vi "Decimate DFD (SANDBOX).vi"(8 "error in (no error)":errorcluster, 10 "Decimation Factor":i32, 11 "Waveforms in":waveform(dbl)[](array[waveform])) -> (0 "error out":errorcluster, 3 "waveforms out":waveform(dbl)[](array[waveform]))   [LabVIEW 2019, in "Instrument.Lockin.lvlib" / "Instrument.DAQ.lvclass"]
uses:
  <vilib>/addons/Digital Filter Design/_Objects.llb/DFD Multirate Filtering Mode.ctl
  <vilib>/Analysis/2dsp.llb/Decimate (single shot, DBL).vi
  Instrument.DAQ.lvclass
  <vilib>/addons/Digital Filter Design/NI_DigFilterLicensed.lvlib
  <vilib>/addons/Digital Filter Design/_Objects.llb/DFD Multirate Filter Specification (Design).ctl
  <vilib>/Analysis/NI_AALPro.lvlib
  <vilib>/measure/NI_MAPro.lvlib
  <vilib>/addons/Digital Filter Design/_Objects.llb/DFD Filter Ripple Specification (Design).ctl
  <vilib>/measure/maresamp.llb/Resample N Waveforms (continuous).vi
  <vilib>/addons/Digital Filter Design/Multirate.llb/DFD NStage MRate Filtering for Single Block (Wfm).vi
  <vilib>/addons/Digital Filter Design/Multirate.llb/DFD NStage MRate Filtering (Wfm).vi
  <vilib>/addons/Digital Filter Design/Multirate.llb/DFD MRate Filtering for Single Block (Wfm NChan).vi
panel:
  out "x != y?":bool
  out "x/y":dbl
  out "Magnitude Response":cluster{"f0":dbl, "df":dbl, "values":dbl[]}[](graph)
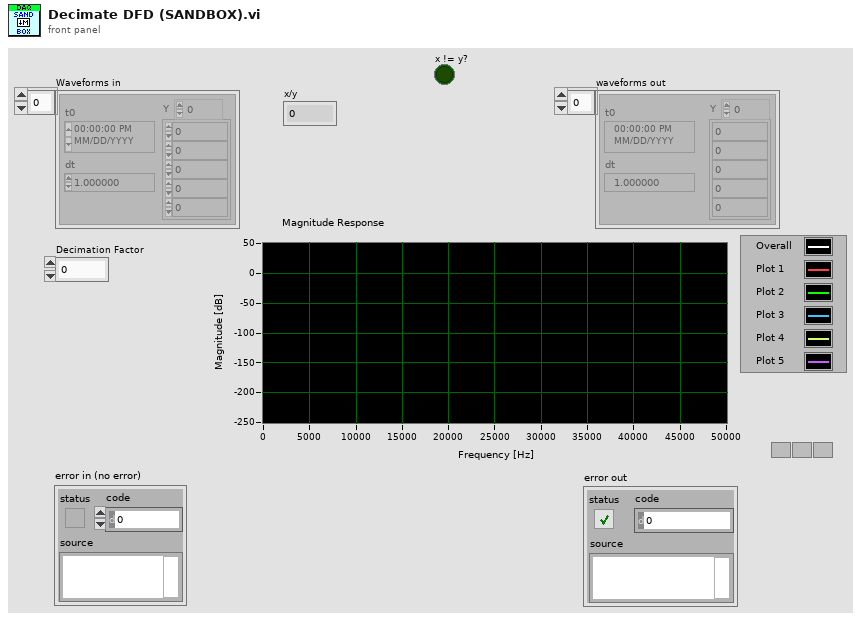
[diagram p1: front panel]
types:
  T1 = typedef "NI_DigFilterLicensed.lvlib/DFD Multirate Filtering Mode.ctl" = u16
  T2 = typedef "NI_DigFilterLicensed.lvlib/DFD Filter Ripple Specification (Design).ctl" = cluster{"passband":dbl, "stopband":dbl, "dB/linear? (T: dB)":bool}
  T3 = typedef "NI_DigFilterLicensed.lvlib/DFD Multirate Filter Specification (Design).ctl" = cluster{"fpass":dbl, "fstop":dbl}
  T4 = typedef "NI_DigFilterLicensed.lvlib/DFD Multirate Filter Obj.ctl" = cluster{"mMRate_Structure":enum16{"CIC", "FIR", "IIR", "Lattice"}, "mMRate_Mode":T5, "mMRate_Factor":i32, "mMRate_FIRParams":cluster{"mMRate_FIR_H":dbl[], "mMRate_FIR_IsNyquist?":bool, "mMRate_FIR_IsSymmetric?":bool}, "mMRate_CICParams":cluster{"mMRate_CIC_#Stage":i32, "mMRate_CIC_Lag":i32, "mMRate_CIC_Type":enum16{"Lowpass", "Highpass"}}, "mMRate_Order":i32, "mMRate_Version":string, "mMRate_Comments":string, "mMRate_RationalFactor":cluster{"mMRate_L":i32, "mMRate_M":i32}, "mMRate_Fs":dbl, "mMRate_Quantized?":bool, "mMRate_QFilterGain":dbl, "mMRate_CoefWl":i16, "mMRate_Scaling":cluster{"mMRate_ScaleByPowerOf2?":bool, "mMRate_ScaleType":T6}, "mMRate_InputWl":i16, "mMRate_OutputWl":i16, "mMRate_OutputMode":T7, "mMRate_MultMode":T8, "mMRate_BitPruning":bool, "mMRate_GainWl":i16, "mMRate_OutputFwl":i16, "mMRate_SumIwl":i16, "mMRate_InputIwl ":i16, "mMRate_SumWl":i16, "mMRate_CoefIwl":i16}
  T5 = typedef "NI_DigFilterLicensed.lvlib/DFD Multirate Mode.ctl" = i16
  T6 = typedef "NI_DigFilterLicensed.lvlib/DFD Coef Norm Type.ctl" = enum16{"No Norm", "Time Domain 1-Norm", "Time Domain 2-Norm", "Time Domain Inf-Norm"}
  T7 = typedef "NI_DigFilterLicensed.lvlib/DFD Round-off Mode.ctl" = enum16{"Nearest", "Truncation"}
  T8 = typedef "NI_DigFilterLicensed.lvlib/DFD FXP MRate Multiply Mode.ctl" = enum16{"Truncated", "Full"}
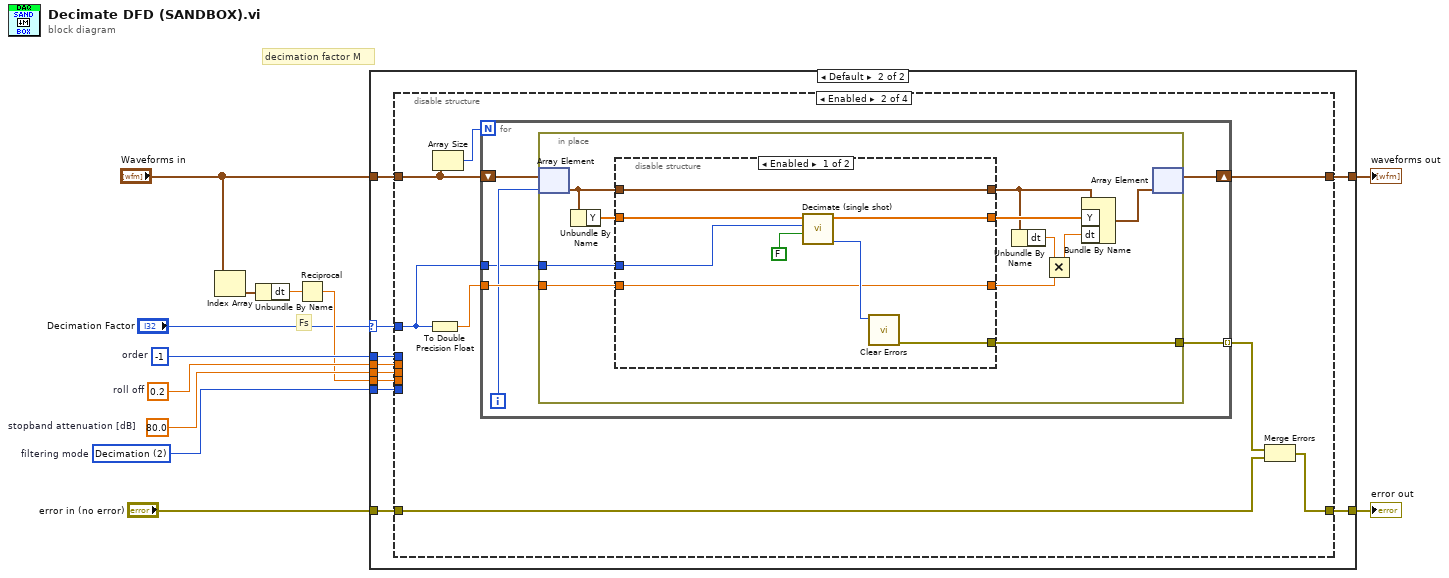
[diagram p0: block diagram]
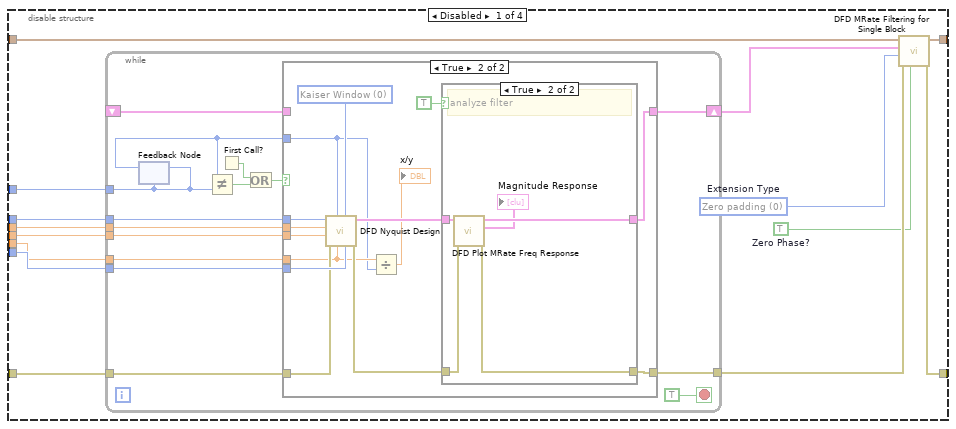
[diagram p3: hidden frame]
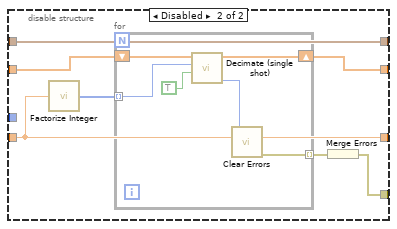
[diagram p6: hidden frame]
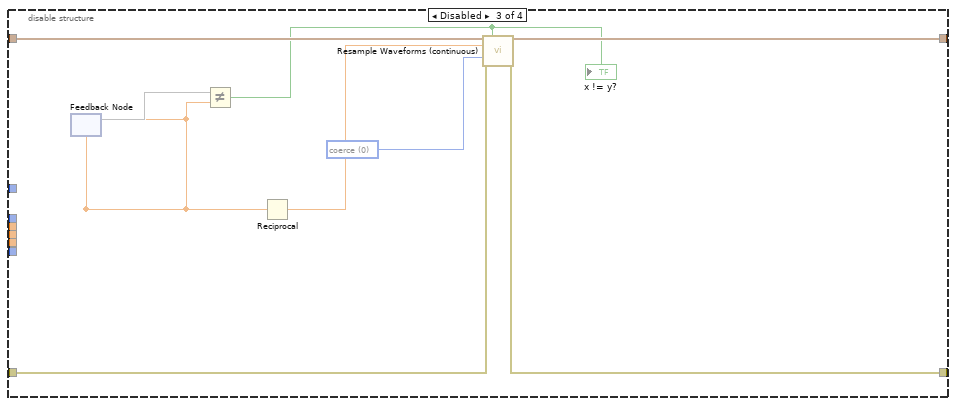
[diagram p7: hidden frame]
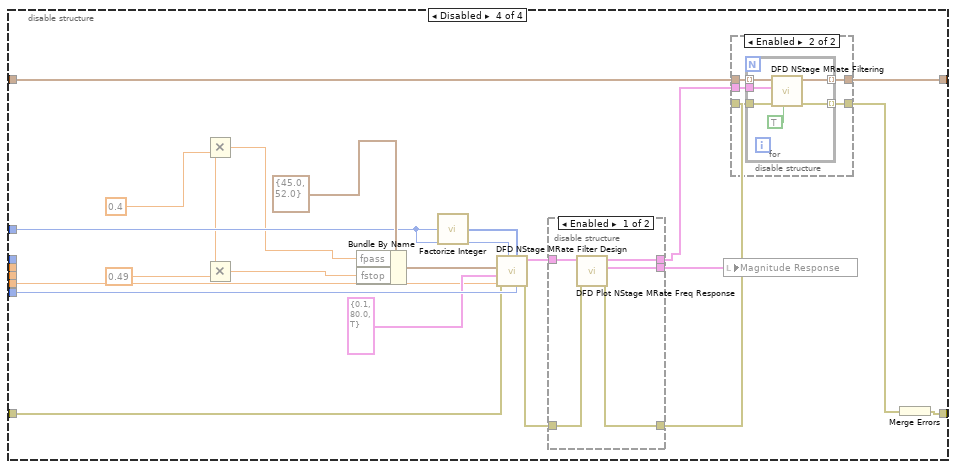
[diagram p8: hidden frame]
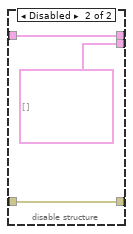
[diagram p9: hidden frame]
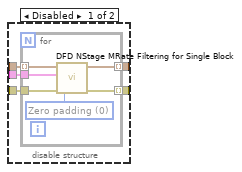
[diagram p10: hidden frame]
diagram:
  w11 = -1  # order
  w9 = 80.0  # stopband attenuation [dB]
  w10 = T1 2 items=["No Rate Change", "Interpolation", "Decimation"]  # filtering mode
  w12 = 0.2  # roll off
  # "Fs"
  # "decimation factor M"
  n1 = Index Array(array="Waveforms in") -> (element=w7:waveform(dbl))  [unwired: 1 in]
  n2 = Unbundle By Name(w7) -> ("dt"=w3:dbl)
  n3 = Reciprocal(x=w3) -> (1/x=w2:dbl)
  n4 = case shown="Default" "Decimation Factor" {
    selector: "Decimation Factor" -> [_ w18]
    tunnel: w12 -> [_ w24]
    tunnel: w10 -> [_ w23]
    tunnel: w9 -> [_ w22]
    tunnel: w11 -> [_ w21]
    tunnel: "Waveforms in" -> [w14 w17]
    tunnel: [w14 w20] -> w8
    tunnel: w2 -> [_ w19]
    tunnel: [w13 w16] -> w5
    tunnel: "error in (no error)" -> [w13 w15]
    frame 0, 1 {
    }
    frame Default {
      n5 = disable-structure shown="Enabled" {
        disable-tunnel: w24 -> [w38 _ _ _]
        disable-tunnel: w23 -> [w37 _ _ w152]
        disable-tunnel: w22 -> [w36 _ _ _]
        disable-tunnel: w21 -> [w35 _ _ _]
        disable-tunnel: [w34 w82 w130 w151] -> w20
        disable-tunnel: w19 -> [w33 _ _ w132]
        disable-tunnel: w17 -> [w30 w80 w131 w135]
        disable-tunnel: w18 -> [w29 w77 _ w143]
        disable-tunnel: [w28 w83 w128 w144] -> w16
        disable-tunnel: w15 -> [w25 w84 w129 w147]
        frame Disabled {
          w26 = TRUE  # Zero Phase?
          w27 = u16 0 items=["Zero padding", "Symmetric", "Periodic"]  # Extension Type
          n6 = while {
            tunnel: w38 -> [w53]
            tunnel: w37 -> [w52]
            tunnel: w36 -> [w51]
            tunnel: w35 -> [w50]
            tunnel: w33 -> [w49]
            tunnel: [w47] -> w31
            shift-right: [w48] -> w32
            shift-left: _ -> [w45]
            tunnel: w29 -> [w40]
            tunnel: w25 -> [w41]
            stop <- TRUE stop-if-true
            n7 = feedback #1(w40) -> (w39:i32)
            n8 = feedback-in #1(w40) -> ()
            n9 = Not Equal?(x=w39, y=w40) -> (x != y?=w43:bool)
            n10 = First Call?() -> (First Call?: T/F=w44:bool)
            n11 = Or(x=w44, y=w43) -> (x .or. y?=w42:bool)
            n12 = case shown="True" w42 {
              tunnel: w53 -> [_ w69]
              tunnel: w52 -> [_ w68]
              tunnel: w51 -> [_ w67]
              tunnel: w50 -> [_ w66]
              tunnel: w49 -> [_ w58]
              tunnel: [w54 w63] -> w48
              tunnel: [w55 w62] -> w47
              tunnel: w45 -> [w54 _]
              tunnel: w39 -> [_ w57]
              tunnel: w41 -> [w55 w59]
              frame False {
              }
              frame True {
                w65 = u16 0 items=["Kaiser Window", "Dolph-Chebyshev Window", "Equi-Ripple", "Positive Equi-Ripple"] ("method")
                n13 = call <vilib>:"DFD Nyquist Design.vi"("filtering mode"=w68, "method"=w65, "fs in [Hz]"=w58, "factor"=w57, "error in (no error)"=w59, "stopband attenuation [dB]"=w67, "roll off"=w69, "order"=w66) -> ("error out"=w60:errorcluster, "multirate filter out"=w64:T4)  [unwired: 2 out]
                n14 = Divide(x=w58, y=w57) -> (x/y=→"x/y":dbl)
                n15 = case shown="True" TRUE {
                  tunnel: w64 -> [w71 w76]
                  tunnel: w60 -> [w70 w73]
                  tunnel: [w71 w75] -> w63
                  tunnel: [w70 w72] -> w62
                  frame False {
                  }
                  frame True {
                    # "analyze filter"
                    n16 = call <vilib>:"DFD Plot MRate Freq Response.vi"("error in (no error)"=w73, "multirate filter in"=w76) -> ("error out"=w72:errorcluster, "magnitude response"=→"Magnitude Response":cluster{"f0":dbl, "df":dbl, "values":dbl[]}[], "multirate filter out"=w75:T4)  [unwired: 5 in, 2 out]
                  }
                }
              }
            }
          }
          n17 = call-poly <vilib>:"DFD MRate Filtering for Single Block.vi"("zero phase? (T)"=w26, "error in (no error)"=w31, "extension type"=w27, "multirate filter"=w32, "signal in"=w30) -> ("error out"=w28:errorcluster, "signal out"=w34:waveform(dbl)[])  [unwired: 5 out]
        }
        frame Enabled {
          n18 = To Double Precision Float(number=w77) -> (double precision float=w78:dbl)
          n19 = Array Size(array=w80) -> (size(s)=w79:i32)
          n20 = for {
            N: w79 -> [_]
            tunnel: w78 -> [w90]
            tunnel: [w89] -> w81 mode=indexing
            shift-right: [w86] -> w82
            shift-left: w80 -> [w88]
            tunnel: w77 -> [w85]
            i -> [w87]
            n21 = in-place {
              in-place-border: w90 -> [w100]
              in-place-border: [w99] -> w89
              in-place-border: w85 -> [w91]
              n22 = in-place-array #2(w88, w87) -> (w93:waveform(dbl))
              n23 = Unbundle By Name(w93) -> ("Y"=w101:dbl[])
              n24 = disable-structure shown="Enabled" {
                disable-tunnel: w101 -> [w109 w116]
                disable-tunnel: w93 -> [w105 w112]
                disable-tunnel: [w105 w112] -> w97
                disable-tunnel: w100 -> [w103 w110]
                disable-tunnel: [w107 w113] -> w99
                disable-tunnel: [w104 w111] -> w98
                disable-tunnel: [w103 w110] -> w95
                disable-tunnel: w91 -> [w102 _]
                frame Enabled {
                  n25 = call-poly <vilib>:"Decimate (single shot).vi"("averaging"=FALSE, "decimating factor"=w102, "X"=w109) -> ("error"=w108:i32, "Decimated Array"=w104:dbl[])  [unwired: 7 in]
                  n26 = call <vilib>:"Clear Errors.vi"("specific error code to clear (0: all)"=w108) -> ("error out"=w107:errorcluster)  [unwired: 5 in, 1 out]
                }
                frame Disabled {
                  n27 = call "Factorize Integer.vi"("Integer in"=w110) -> ("Integer Factors"=w115:i32[])
                  n28 = for {
                    shift-right: [w121] -> w111
                    shift-left: w116 -> [w122]
                    tunnel: w115 -> [w120] mode=indexing
                    tunnel: [w117] -> w114 mode=indexing
                    n29 = call-poly <vilib>:"Decimate (single shot).vi"("averaging"=TRUE, "decimating factor"=w120, "X"=w122) -> ("error"=w118:i32, "Decimated Array"=w121:dbl[])  [unwired: 7 in]
                    n30 = call <vilib>:"Clear Errors.vi"("specific error code to clear (0: all)"=w118) -> ("error out"=w117:errorcluster)  [unwired: 5 in, 1 out]
                  }
                  n31 = Merge Errors(w114) -> (w113:errorcluster)
                }
              }
              n32 = Unbundle By Name(w97) -> ("dt"=w96:dbl)
              n33 = Multiply(x=w96, y=w95) -> (x*y=w94:dbl)
              n34 = Bundle By Name(cluster=w97, "Y"=w98, "dt"=w94) -> (w92:waveform(dbl))
              n35 = in-place-array #2(w92) -> (w86:waveform(dbl)[])  [unwired: 1 out]
            }
          }
          n36 = Merge Errors(w81, w84) -> (w83:errorcluster)
        }
        frame Disabled {
          w123 = u16 0 items=["coerce", "linear", "spline", "FIR filter"] ("interpolation mode")
          n37 = Reciprocal() -> (x=w125:dbl, 1/x=w127:dbl)
          n38 = feedback #3(w125) -> (w126)
          n39 = feedback-in #3(w125) -> ()
          n40 = Not Equal?(x=w126, y=w125) -> (x != y?=w124:bool)
          "x != y?" <- w124
          n41 = call-poly <vilib>:"Resample Waveforms (continuous).vi"("waveforms in"=w131, "reset"=w124, "dt"=w127, "interpolation mode"=w123, "error in (no error)"=w129) -> ("resampled waveforms out"=w130:waveform(dbl)[], "error out"=w128:errorcluster)  [unwired: 6 in, 3 out]
        }
        frame Disabled {
          n42 = Multiply(y=0.49) -> (x=w140:dbl, x*y=w134:dbl)
          n43 = Multiply(x=w140, y=0.4) -> (x*y=w139:dbl)
          n44 = Bundle By Name(cluster=T3 {"fpass"=45.0, "fstop"=52.0} ("freq specs [Hz]"), "fpass"=w139, "fstop"=w134) -> (w148:T3)
          n45 = call "Factorize Integer.vi"("Integer in"=w143) -> ("Integer Factors"=w133:i32[])
          n46 = call <vilib>:"DFD NStage MRate Filter Design.vi"("filtering mode"=w152, "manual factorization"=w133, "fs in [Hz]"=w132, "factor"=w143, "error in (no error)"=w147, "ripple specs"=T2 {"passband"=0.1, "stopband"=80.0, "dB/linear? (T: dB)"=TRUE}, "freq specs [Hz]"=w148) -> ("error out"=w142:errorcluster, "multirate filters out"=w145:T4[])  [unwired: 3 in]
          n47 = disable-structure shown="Enabled" {
            disable-tunnel: [w158 cluster{"f0":dbl, "df":dbl, "values":dbl[]}[] [] ("Magnitude Response")] -> w153
            disable-tunnel: w145 -> [w157 w161]
            disable-tunnel: [w156 w161] -> w136
            disable-tunnel: w142 -> [w155 w160]
            disable-tunnel: [w154 w160] -> w141
            frame Enabled {
              n48 = call <vilib>:"DFD Plot NStage MRate Freq Response.vi"("error in (no error)"=w155, "multirate filters in"=w157) -> ("error out"=w154:errorcluster, "magnitude responses"=w158:cluster{"f0":dbl, "df":dbl, "values":dbl[]}[], "multirate filters out"=w156:T4[])  [unwired: 6 in, 1 out]
            }
            frame Disabled {
            }
          }
          n49 = local write "Magnitude Response"(w153) -> ()
          n50 = disable-structure shown="Enabled" {
            disable-tunnel: [w166 w176] -> w151
            disable-tunnel: [w165 w173] -> w146
            disable-tunnel: w141 -> [w164 w174]
            disable-tunnel: w135 -> [w163 w177]
            disable-tunnel: w136 -> [w162 w175]
            frame Disabled {
              n51 = for {
                tunnel: w163 -> [w172] mode=indexing
                tunnel: w162 -> [w171]
                tunnel: [w170] -> w166 mode=indexing
                tunnel: w164 -> [w168]
                tunnel: [w167] -> w165 mode=indexing
                w169 = u16 0 items=["Zero padding", "Symmetric", "Periodic"] ("extension type")
                n52 = call-poly <vilib>:"DFD NStage MRate Filtering for Single Block.vi"("error in (no error)"=w168, "extension type"=w169, "multirate filters"=w171, "signal in"=w172) -> ("error out"=w167:errorcluster, "signal out"=w170:waveform(dbl))  [unwired: 6 in]
              }
            }
            frame Enabled {
              n53 = for {
                tunnel: w177 -> [w183] mode=indexing
                tunnel: [w182] -> w176 mode=indexing
                tunnel: w175 -> [w181]
                tunnel: w174 -> [w179]
                tunnel: [w178] -> w173 mode=indexing
                n54 = call-poly <vilib>:"DFD NStage MRate Filtering.vi"("zero phase? (T)"=TRUE, "error in (no error)"=w179, "multirate filters"=w181, "signal in"=w183) -> ("error out"=w178:errorcluster, "signal out"=w182:waveform(dbl))  [unwired: 1 in, 5 out]
              }
            }
          }
          n55 = Merge Errors(w146) -> (w144:errorcluster)
        }
      }
    }
  }
  "waveforms out" <- w8
  "error out" <- w5
